vi "Move_Rel_FullBit.vi"(2 "relative Z":dbl, 3 "handle":i32) -> ()   [LabVIEW 2020]
uses:
  Dependencies/Madlib.dll
panel:
  out "x*y":dbl
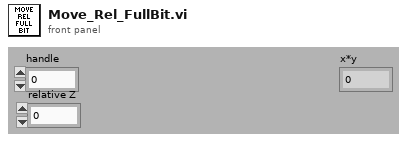
[diagram p1: front panel]
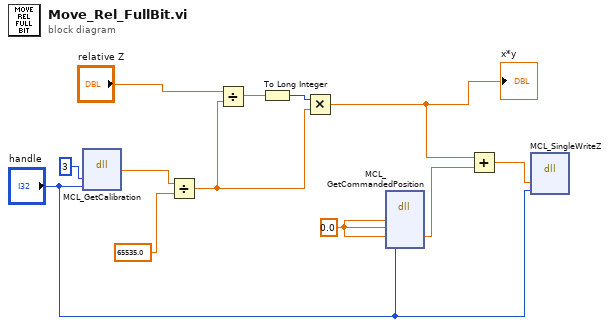
[diagram p0: block diagram]
diagram:
  w6 = 0.0 ("commandX")
  n1 = dll-call lib="D:/Daguan/Development/RM21-MMicrosopeSource/HardwareAdapter/Stages/Dependencies/Madlib.dll" fn="MCL_GetCalibration"("axis"=u32 3, "handle"="handle") -> ("size"=w12:dbl)  [unwired: 5 in, 2 out]
  n2 = Divide(x=w12, y=65535.0) -> (x/y=w7:dbl)
  n3 = Divide(x="relative Z", y=w7) -> (x/y=w9:dbl)
  n4 = To Long Integer(number=w9) -> (32bit integer=w8:i32)
  n5 = Multiply(x=w8, y=w7) -> (x*y=w2:dbl)
  "x*y" <- w2
  n6 = dll-call lib="D:/Daguan/Development/RM21-MMicrosopeSource/HardwareAdapter/Stages/Dependencies/Madlib.dll" fn="MCL_GetCommandedPosition" label="MCL_SingleReadN"("commandX"=w6, "commandY"=w6, "commandZ"=w6, "handle"="handle") -> ("commandZ"=w1:dbl)  [unwired: 5 in, 4 out]
  n7 = Add(x=w2, y=w1) -> (x+y=w3:dbl)
  n8 = dll-call lib="D:/Daguan/Development/RM21-MMicrosopeSource/HardwareAdapter/Stages/Dependencies/Madlib.dll" fn="MCL_SingleWriteZ"("position"=w3, "handle"="handle") -> ()  [unwired: 3 in, 5 out]
